vi "LoadAutoConfig.vi"(11 "file path (dialog if empty)":path) -> (0 "error out":errorcluster, 1 "Times":i64[](array[numeric]), 2 "Turbine RPMs":i64[](array[numeric]), 3 "Pump RPMs":i64[](array[numeric]))   [LabVIEW 2024, in "UI.lvlib"]
uses:
  UI.lvlib
  <vilib>/Utility/file.llb/Read Delimited Spreadsheet (I64).vi
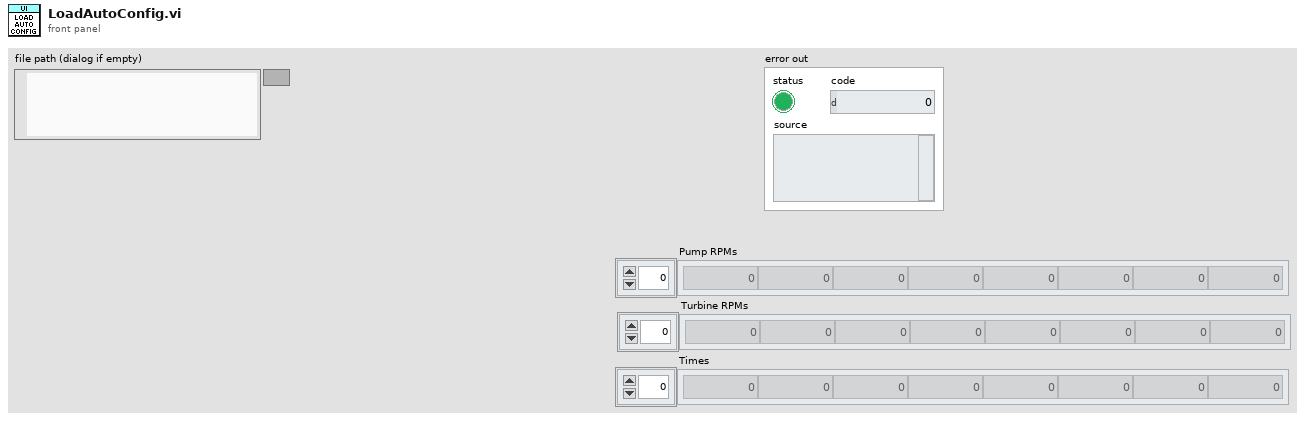
[diagram p1: front panel]
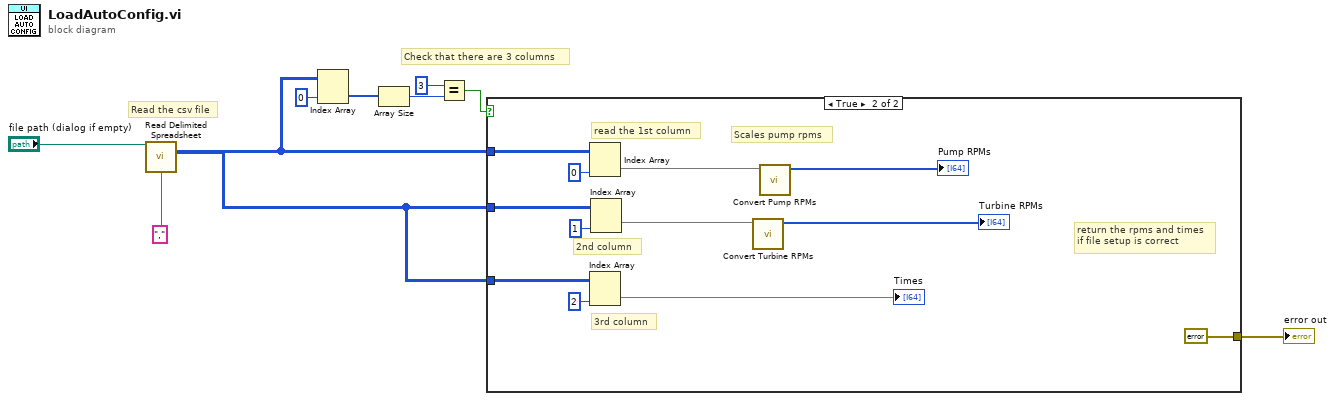
[diagram p0: block diagram]
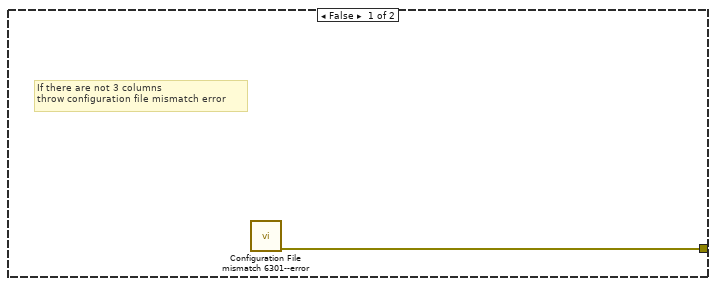
[diagram p2: hidden frame]
diagram:
  # "Check that there are 3 columns"
  # "Read the csv file"
  n1 = call-poly <vilib>:"Read Delimited Spreadsheet.vi"("file path (dialog if empty)"="file path (dialog if empty)", "delimiter (\\t)"="," ("delimiter (\\t)")) -> ("all rows"=w1:i64[][])  [unwired: 8 in, 5 out]
  n2 = Index Array(array=w1, index (row)=0) -> (element=w5:i64[])  [unwired: 1 in]
  n3 = Array Size(array=w5) -> (size(s)=w4:i32)
  n4 = Equal?(x=3, y=w4) -> (x = y?=w2:bool)
  n5 = case shown="True" w2 {
    tunnel: [w10 errorcluster {"status"=FALSE, "code"=0, "source"=""} ("error out")] -> w7
    tunnel: w1 -> [_ w19]
    tunnel: w1 -> [_ w17]
    tunnel: w1 -> [_ w15]
    frame False {
      # "If there are not 3 columns\nthrow configuration file mismatch error"
      n6 = call "Configuration File mismatch 6301--error.vi"() -> ("error out"=w10:errorcluster)  [unwired: 11 in]
    }
    frame True {
      # "Scales pump rpms"
      # "2nd column"
      # "3rd column"
      # "read the 1st column"
      # "return the rpms and times\nif file setup is correct"
      n7 = Index Array(array=w15, index (col)=0 ("disabled index (col)")) -> (element=w20:i64[])  [unwired: 1 in]
      n8 = Index Array(array=w19, index (col)=2 ("disabled index (col)")) -> (element=→"Times":i64[])  [unwired: 1 in]
      n9 = Index Array(array=w17, index (col)=1 ("disabled index (col)")) -> (element=w21:i64[])  [unwired: 1 in]
      n10 = call "Convert Turbine RPMs.vi"("RPMs input"=w21) -> ("RPMs Output"=→"Turbine RPMs":i64[])  [unwired: 10 in]
      n11 = call "Convert Pump RPMs.vi"("RPMs input"=w20) -> ("RPMs Output"=→"Pump RPMs":i64[])  [unwired: 10 in]
    }
  }
  "error out" <- w7
